vi "Check limit.vi"() -> ()   [LabVIEW 2013]
panel:
  in  "String":string="发射点感67685xcz "
  out "string":string
  out "first char last":string
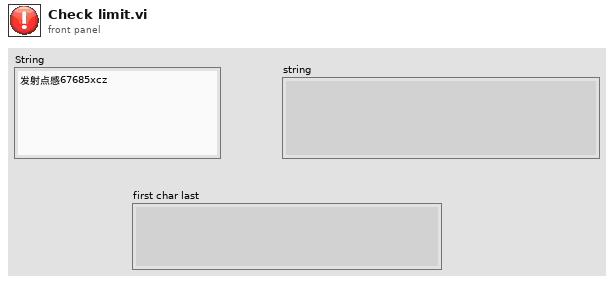
[diagram p1: front panel]
types:
  T1 = enum16{"open", "replace", "create", "open or create", "replace or create", "replace or create with confirmation"}
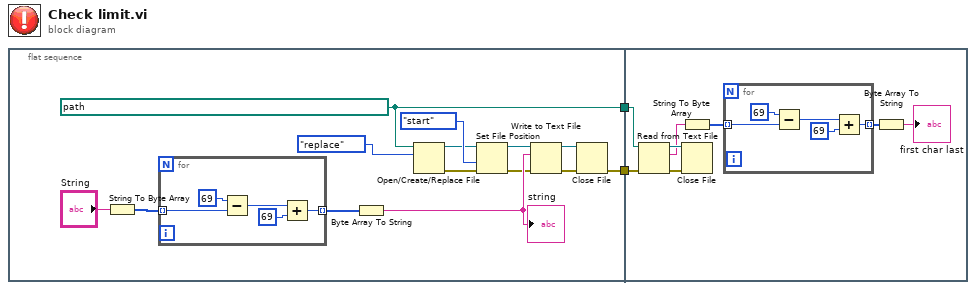
[diagram p0: block diagram]
diagram:
  n1 = flat-sequence {
    tunnel: [w4] -> w2
    tunnel: [w14] -> w1
    tunnel: w2 -> [w29]
    tunnel: w1 -> [w28]
    frame #0 {
      w14 = path "E:/My Project/松虹电子/Converted/Configure/SystemSetting.ini" ("file path (use dialog)")
      n2 = String To Byte Array(string="String") -> (unsigned byte array=w13:u8[])
      n3 = for {
        tunnel: w13 -> [w20] mode=indexing
        tunnel: [w17] -> w12 mode=indexing
        n4 = Subtract(x=u8 69, y=w20) -> (x-y=w19:u8)
        n5 = Add(x=w19, y=u8 69) -> (x+y=w17:u8)
      }
      n6 = Byte Array To String(unsigned byte array=w12) -> (string=w10:string)
      "string" <- w10
      n7 = Open/Create/Replace File(file path (use dialog)=w14, operation (0:open)=T1."replace") -> (refnum out=w8:refnum<file>, error out=w6:errorcluster)  [unwired: 4 in, 1 out]
      n8 = Set File Position(refnum=w8, from (0:start)=enum16{"start", "end", "current"}."start", error in=w6) -> (refnum out=w7:refnum<file>, error out=w5:errorcluster)  [unwired: 1 in]
      n9 = Write to Text File(file (use dialog)=w7, text=w10, error in=w5) -> (refnum out=w15:refnum<file>, error out=w16:errorcluster)  [unwired: 1 in, 1 out]
      n10 = Close File(refnum=w15, error in=w16) -> (error out=w4:errorcluster)  [unwired: 1 out]
    }
    frame #1 {
      n11 = Read from Text File(file (use dialog)=w28, error in=w29) -> (refnum out=w26:refnum<file>, text=w23:string, error out=w27:errorcluster)  [unwired: 2 in, 1 out]
      n12 = String To Byte Array(string=w23) -> (unsigned byte array=w24:u8[])
      n13 = Close File(refnum=w26, error in=w27) -> ()  [unwired: 2 out]
      n14 = for {
        tunnel: w24 -> [w33] mode=indexing
        tunnel: [w30] -> w25 mode=indexing
        n15 = Subtract(x=u8 69, y=w33) -> (x-y=w32:u8)
        n16 = Add(x=w32, y=u8 69) -> (x+y=w30:u8)
      }
      n17 = Byte Array To String(unsigned byte array=w25) -> (string=→"first char last":string)
    }
  }
